vi "WrapPhase.vi"(11 "phase (upwrapped)":dbl[](array[numeric])) -> (3 "phase (wrapped)":dbl[](array[numeric]))   [LabVIEW 2022 SP3]
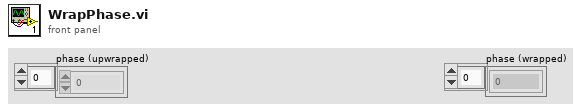
[diagram p1: front panel]
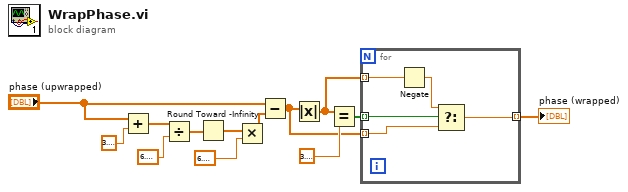
[diagram p0: block diagram]
diagram:
  n1 = Add(x="phase (upwrapped)", y=3.141592653589793) -> (x+y=w11:dbl[])
  n2 = Divide(x=w11, y=6.283185307179586) -> (x/y=w9:dbl[])
  n3 = Round Toward -Infinity(1:w9) -> (0:w8:dbl[])
  n4 = Multiply(x=w8, y=6.283185307179586) -> (x*y=w6:dbl[])
  n5 = Subtract(x="phase (upwrapped)", y=w6) -> (x-y=w1:dbl[])
  n6 = Absolute Value(x=w1) -> (abs(x)=w4:dbl[])
  n7 = Equal?(x=w4, y=3.141592653589793) -> (x = y?=w3:bool[])
  n8 = for {
    tunnel: w4 -> [w16] mode=indexing
    tunnel: w3 -> [w18] mode=indexing
    tunnel: [w15] -> w2 mode=indexing
    tunnel: w1 -> [w14] mode=indexing
    n9 = Negate(x=w16) -> (-x=w17:dbl)
    n10 = Select(t=w17, s=w18, f=w14) -> (s? t:f=w15:dbl)
  }
  "phase (wrapped)" <- w2
